vi "sendStop.vi"(8 "error in (no error)":errorcluster, 10 "stop":enum16{"stopBeforeNext", "stopNow"}(ring), 11 "ExperimentRunner in":refnum<class "ExperimentRunner.lvclass">) -> (0 "error out":errorcluster, 3 "ExperimentRunner out":refnum<class "ExperimentRunner.lvclass">)   [LabVIEW 2009, in "Views.lvlib" / "ExperimentControl.lvlib" / "ExperimentRunner.lvclass"]
uses:
  ExperimentRunner.lvclass
  ExperimentRunner.lvclass/ExperimentRunner.ctl
  Events/ExperimentControlEvents.lvclass
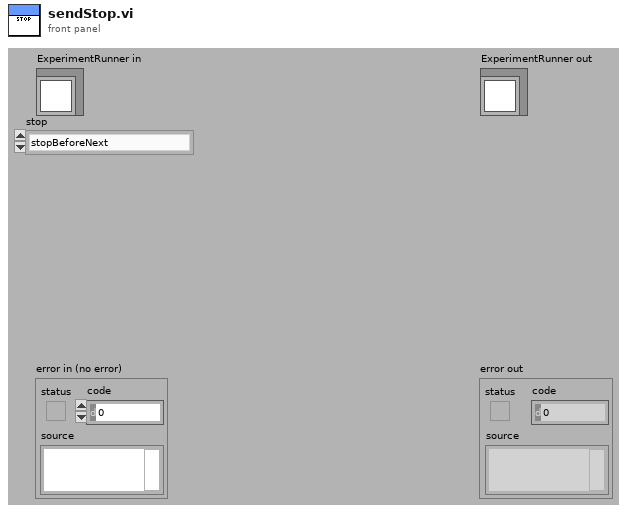
[diagram p1: front panel]
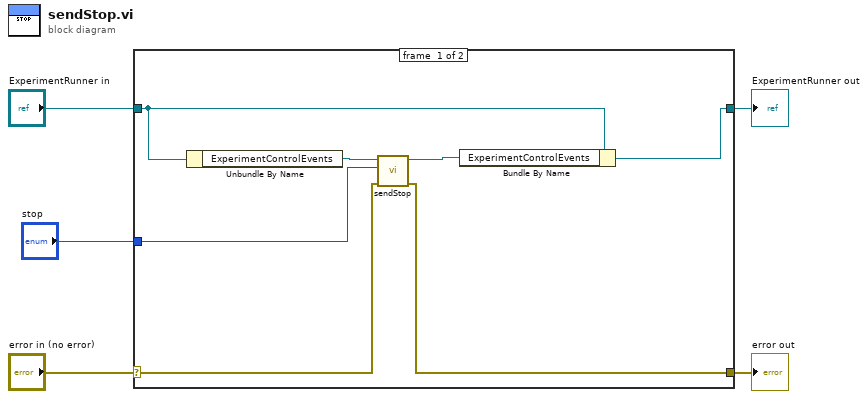
[diagram p0: block diagram]
diagram:
  n1 = case shown="No Error" "error in (no error)" {
    selector: "error in (no error)" -> [w10 w14]
    tunnel: [w11 w14] -> w4
    tunnel: [w6 w13] -> w2
    tunnel: "ExperimentRunner in" -> [w8 w13]
    tunnel: "stop" -> [w9 _]
    frame #0 {
      n2 = Unbundle By Name(w8) -> ("ExperimentControlEvents"=w12:refnum<class "ExperimentControlEvents.lvclass">)
      n3 = call "sendStop.vi"("error in (no error)"=w10, "stop"=w9, "ExperimentControlEvents in"=w12) -> ("error out"=w11:errorcluster, "ExperimentControlEvents out"=w7:refnum<class "ExperimentControlEvents.lvclass">)  [unwired: 7 in]
      n4 = Bundle By Name(cluster=w8, "ExperimentControlEvents"=w7) -> (w6:refnum<class "ExperimentRunner.lvclass">)
    }
    frame #1 {
    }
  }
  "error out" <- w4
  "ExperimentRunner out" <- w2
